vi "Write write_.vi"(8 "error in (no error)":errorcluster, 10 "write?":bool, 11 "Set Write Ringdowns CMD in":refnum<class "Set Write Ringdowns CMD.lvclass">) -> (0 "error out":errorcluster, 3 "Set Write Ringdowns CMD out":refnum<class "Set Write Ringdowns CMD.lvclass">)   [LabVIEW 2014, in "eCRDS Library.lvlib" / "Set Write Ringdowns CMD.lvclass"]
uses:
  Set Write Ringdowns CMD.lvclass
  Set Write Ringdowns CMD.lvclass/Set Write Ringdowns CMD.ctl
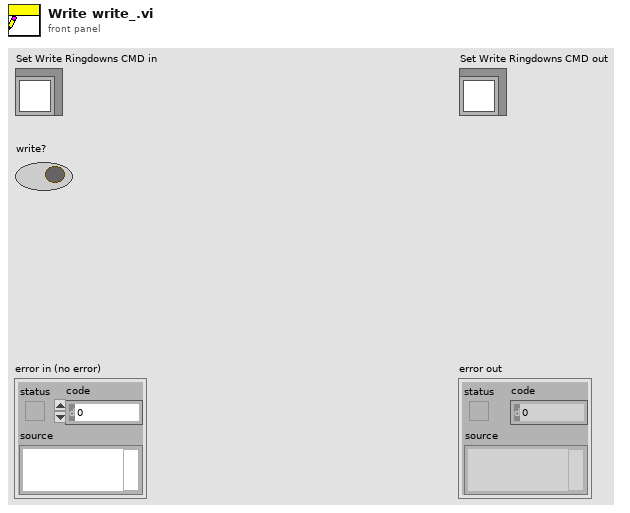
[diagram p1: front panel]
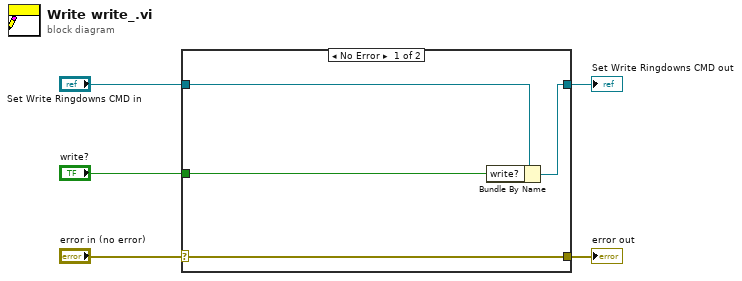
[diagram p0: block diagram]
diagram:
  n1 = case shown="No Error" "error in (no error)" {
    selector: "error in (no error)" -> [w9 w10]
    tunnel: [w9 w10] -> w4
    tunnel: [w7 w11] -> w2
    tunnel: "Set Write Ringdowns CMD in" -> [w8 w11]
    tunnel: "write?" -> [w6 _]
    frame No Error {
      n2 = Bundle By Name(cluster=w8, "write?"=w6) -> (w7:refnum<class "Set Write Ringdowns CMD.lvclass">)
    }
    frame Error {
    }
  }
  "error out" <- w4
  "Set Write Ringdowns CMD out" <- w2
